vi "Open Topic Lookup Table Reference.vi"(8 "error in (no error)":errorcluster, 11 "TopicLookupTable in":refnum<class "TopicLookupTable.lvclass">) -> (0 "error out":errorcluster, 3 "TopicLookupTable Reference":refnum<data-value>)   [LabVIEW 2020, in "Mediator.lvlib" / "TopicLookupTable.lvclass"]
uses:
  <vilib>/gpm_packages/@cs/mva-core/Source/Mediator/TopicLookupTable/TopicLookupTable.lvclass
panel:
  # "Optional input, useful only if special types\nof TopicLookupTables exist (no subtypes\nexist at the time of this comment)."
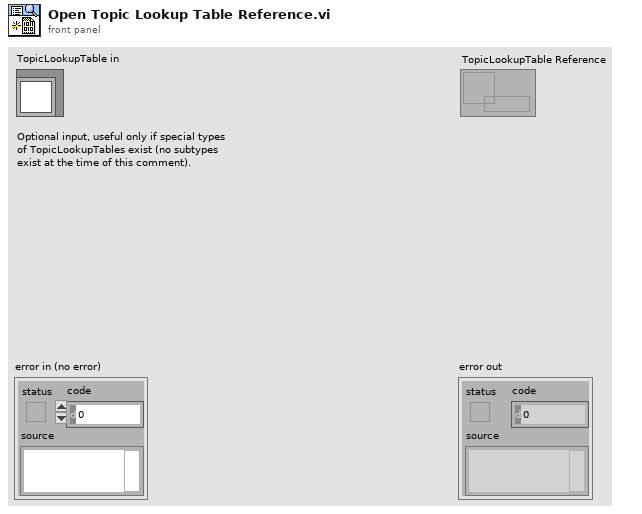
[diagram p1: front panel]
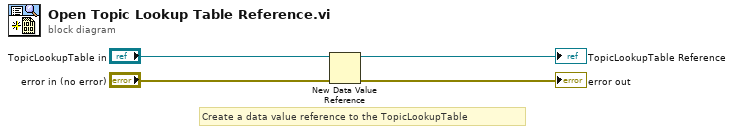
[diagram p0: block diagram]
diagram:
  # "Create a data value reference to the TopicLookupTable"
  n1 = New Data Value Reference(data value="TopicLookupTable in", error in="error in (no error)") -> (data value reference=→"TopicLookupTable Reference":refnum<data-value>, error out=→"error out":errorcluster)
